vi "Go to field (immediately) (No Objects).vi"(8 "error in":errorcluster, 10 "Desired field (T)":dbl[unit], 11 "Varian Magnet In":T2={"Fluke VISA resource name"="GPIB0::2::INSTR", "DAQ Physical Channel"="Dev1/ao0", "DAQ Task - Set"="", "DAQ Task - Read"="", "Control Voltage"=enum."40V", "extrapolated"={"x locations"=[], "coefficients"=[]}, "last 5 field numbers"=[], "Fluke Multimeter"={"function (0:volts DC)"=0, "range (0:auto)"=0, "rate (0:slow)"=0, "trigger mode (0:internal)"=0, "Autorange"=FALSE}} {"extrapolated"."x locations" format="%.4g"; "extrapolated"."coefficients" format="%.4g"; "Fluke Multimeter"."function (0:volts DC)" items=["volts DC", "volts AC", "2-wire k.ohms", "4-wire k.ohms", "mA DC", "mA AC"]; "Fluke Multimeter"."range (0:auto)" items=["autorange", "200mV, 200 ohms", "2V, 2 kohms", "20V, 20 kohms", "200V, 200 kohms", "1000Vdc, 700 Vac, 2 Mohms", "20 Mohms"]; "Fluke Multimeter"."rate (0:slow)" items=["slow", "medium", "fast"]; "Fluke Multimeter"."trigger mode (0:internal)" items=["internal - continuous trigger", "external - rear panel trigger with delay", "external - bus trigger with delay", "external - rear panel trigger", "external - bus trigger"]}) -> (0 "error out":errorcluster, 3 "Varian Magnet Out":T2={"Fluke VISA resource name"="GPIB0::2::INSTR", "DAQ Physical Channel"="Dev1/ao0", "DAQ Task - Set"="", "DAQ Task - Read"="", "Control Voltage"=enum."40V", "extrapolated"={"x locations"=[], "coefficients"=[]}, "last 5 field numbers"=[], "Fluke Multimeter"={"function (0:volts DC)"=0, "range (0:auto)"=0, "rate (0:slow)"=0, "trigger mode (0:internal)"=0, "Autorange"=FALSE}} {"extrapolated"."x locations" format="%.4g"; "extrapolated"."coefficients" format="%.4g"; "Fluke Multimeter"."function (0:volts DC)" items=["volts DC", "volts AC", "2-wire k.ohms", "4-wire k.ohms", "mA DC", "mA AC"]; "Fluke Multimeter"."range (0:auto)" items=["autorange", "200mV, 200 ohms", "2V, 2 kohms", "20V, 20 kohms", "200V, 200 kohms", "1000Vdc, 700 Vac, 2 Mohms", "20 Mohms"]; "Fluke Multimeter"."rate (0:slow)" items=["slow", "medium", "fast"]; "Fluke Multimeter"."trigger mode (0:internal)" items=["internal - continuous trigger", "external - rear panel trigger with delay", "external - bus trigger with delay", "external - rear panel trigger", "external - bus trigger"]})   [LabVIEW 2009]
doc: "Sets the control voltage based on the Long-Term Field Calibration in Varian Constants.vi Global."
uses:
  <vilib>/gmath/interp.llb/in_piecewise interp poly control.ctl
  Varian Constants (No Objects).vi
  <vilib>/gmath/NI_Gmath.lvlib
  Varian/Varian.lvlib
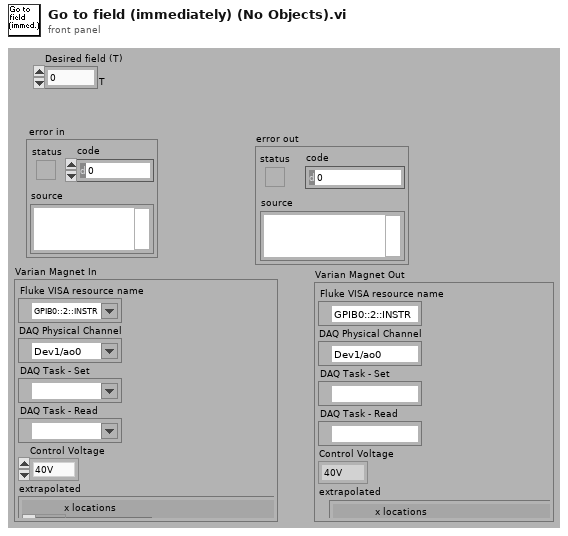
[diagram p1: front panel]
types:
  T1 = typedef "NI_Gmath.lvlib/in_piecewise interp poly control.ctl" = cluster{"x locations":dbl[], "coefficients":dbl[][]}
  T2 = cluster{"Fluke VISA resource name":refnum<visa-resource-name>, "DAQ Physical Channel":tag, "DAQ Task - Set":refnum<k21>, "DAQ Task - Read":refnum<k21>, "Control Voltage":enum16{"Please Select a Value", "30V", "40V"}, "extrapolated":T1, "last 5 field numbers":dbl[], "Fluke Multimeter":cluster{"function (0:volts DC)":u16, "range (0:auto)":u16, "rate (0:slow)":u16, "trigger mode (0:internal)":u16, "Autorange":bool}}
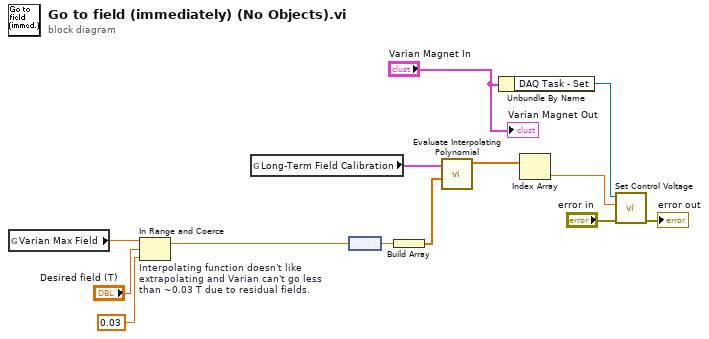
[diagram p0: block diagram]
diagram:
  n1 = global read "Varian Constants (No Objects).vi" "Varian Max Field"() -> (w2:dbl[unit])
  n2 = In Range and Coerce "Interpolating function doesn't like\nextrapolating and Varian can't go less\nthan ~0.03 T due to residual fields."(upper limit=w2, x="Desired field (T)", lower limit=dbl[unit] 0.03) -> (coerced(x)=w6:dbl[unit])  [unwired: 1 out]
  n3 = global read "Varian Constants (No Objects).vi" "Long-Term Field Calibration"() -> (w1:T1)
  n4 = node(w6) -> (w5:dbl)
  n5 = Build Array(w5) -> (w13:dbl[])
  n6 = call <vilib>:"Evaluate Interpolating Polynomial.vi"("xi"=w13, "piecewise polynomial"=w1) -> ("yi"=w12:dbl[])  [unwired: 8 in, 1 out]
  n7 = Unbundle By Name("Varian Magnet In") -> ("DAQ Task - Set"=w11:refnum<k21>)
  n8 = Index Array(array=w12) -> (element=w10:dbl)  [unwired: 1 in]
  n9 = call "Set Control Voltage.vi"("error in"="error in", "Control Voltage"=w10, "task in"=w11) -> ("error out"=→"error out":errorcluster)  [unwired: 7 in, 1 out]
  "Varian Magnet Out" <- "Varian Magnet In"
